vi "Populate Run-Time Menu.vi"(8 "error in (no error)":errorcluster, 10 "Menu in":refnum<k9>, 11 "Execution UI In":refnum<class "Execution UI.lvclass">) -> (0 "error out":errorcluster, 3 "Execution UI Out":refnum<class "Execution UI.lvclass">)   [LabVIEW 2020, in "Execution UI.lvclass"]
uses:
  Execution UI.lvclass
  Execution UI.lvclass/Execution UI.ctl
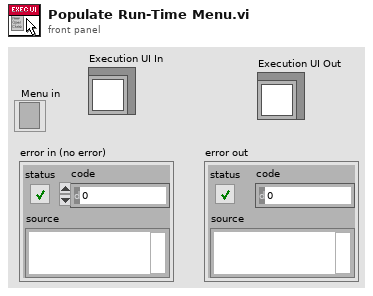
[diagram p1: front panel]
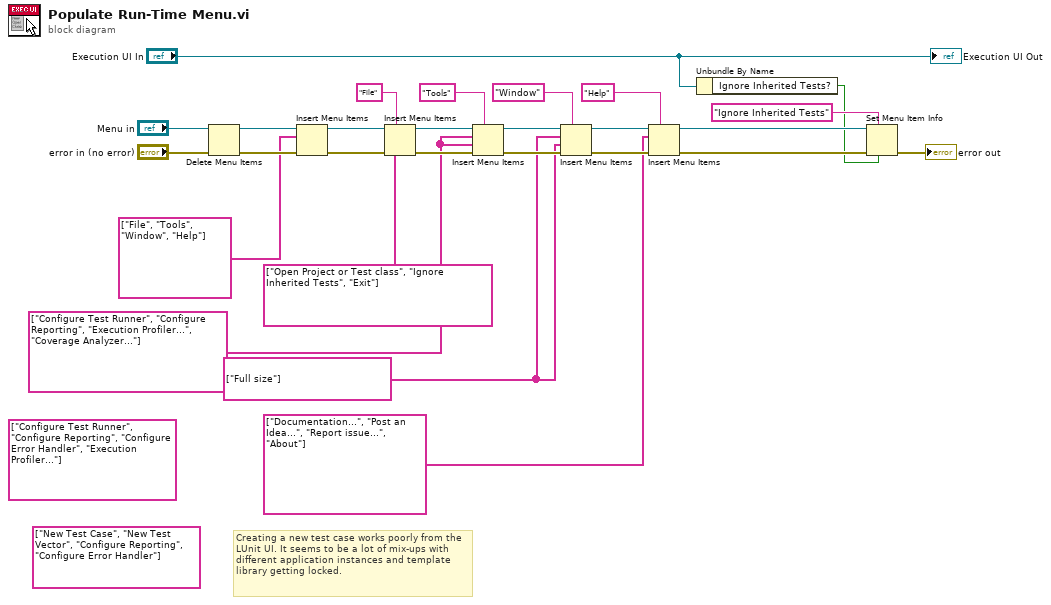
[diagram p0: block diagram]
diagram:
  (unwired) string[] ["Configure Test Runner", "Configure Reporting", "Configure Error Handler", "Execution Profiler..."] ("item names")
  (unwired) string[] ["New Test Case", "New Test Vector", "Configure Reporting", "Configure Error Handler"] ("item names")
  w8 = string[] ["Full size"] ("item names")
  w9 = string[] ["Configure Test Runner", "Configure Reporting", "Execution Profiler...", "Coverage Analyzer..."] ("item names")
  w2 = string[] ["Open Project or Test class", "Ignore Inherited Tests", "Exit"] ("item names")
  # "Creating a new test case works poorly from the LUnit UI. It seems to be a lot of mix-ups with different application instances and template library getting locked."
  n1 = Delete Menu Items(6:"error in (no error)", 9:"Menu in") -> (0:w24:errorcluster, 3:w26:refnum<k9>)  [unwired: 2 in]
  n2 = Insert Menu Items(6:w24, 8:string[] ["File", "Tools", "Window", "Help"] ("item names"), 9:w26) -> (0:w21:errorcluster, 3:w22:refnum<k9>)  [unwired: 3 in, 1 out]
  n3 = Insert Menu Items(5:"File" ("menu tag"), 6:w21, 7:w2, 8:w2, 9:w22) -> (0:w17:errorcluster, 3:w16:refnum<k9>)  [unwired: 1 in, 1 out]
  n4 = Insert Menu Items(5:"Tools", 6:w17, 7:w9, 8:w9, 9:w16) -> (0:w18:errorcluster, 3:w15:refnum<k9>)  [unwired: 1 in, 1 out]
  n5 = Insert Menu Items(5:"Window", 6:w18, 7:w8, 8:w8, 9:w15) -> (0:w19:errorcluster, 3:w14:refnum<k9>)  [unwired: 1 in, 1 out]
  n6 = Insert Menu Items(5:"Help", 6:w19, 8:string[] ["Documentation...", "Post an Idea...", "Report issue...", "About"] ("item names"), 9:w14) -> (0:w6:errorcluster, 3:w7:refnum<k9>)  [unwired: 2 in, 1 out]
  n7 = Unbundle By Name("Execution UI In") -> ("Ignore Inherited Tests?"=w1:bool)
  n8 = Set Menu Item Info(6:w1, 7:"Ignore Inherited Tests", 8:w6, 11:w7) -> (0:→"error out":errorcluster)  [unwired: 3 in, 1 out]
  "Execution UI Out" <- "Execution UI In"
